vi "PDU Init.vi"(8 "error in (no error)":errorcluster, 10 "Name":string, 11 "Orion PDU in":refnum<class "Orion PDU.lvclass">) -> (0 "error out":errorcluster, 3 "Orion PDU out":refnum<class "Orion PDU.lvclass">)   [LabVIEW 2022 SP3, in "Orion PDU.lvclass"]
uses:
  Orion PDU.lvclass
  C:/Development/rimas/RIMAS/Power Distribution/Power Distribution.lvclass
  Power Distribution.lvclass/Power Distribution.ctl
  Orion PDU.lvclass/Orion PDU.ctl
  Power Distribution.lvclass
  <vilib>/httpClient/LabVIEWHTTPClient.lvlib
panel:
  # "rimas pdu1"
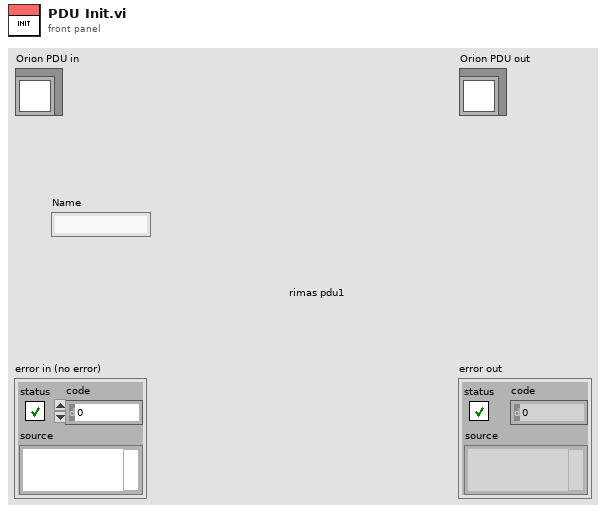
[diagram p1: front panel]
types:
  T1 = typedef "Orion PDU.lvclass/typedef Orion PDU Settings.ctl" = cluster{"URL":string, "Username":string, "Password":string}
  T2 = typedef "LabVIEWHTTPClient.lvlib/ClientHandle.ctl" = refnum<k1>
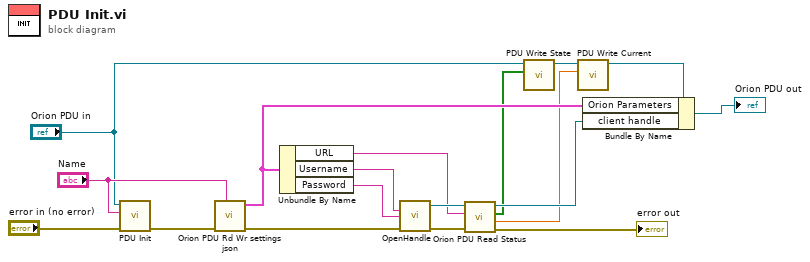
[diagram p0: block diagram]
diagram:
  n1 = call-parent "PDU Init.vi"("error in (no error)"="error in (no error)", "Name"="Name", "Power Distribution in"="Orion PDU in") -> ("error out"=w17:errorcluster)  [unwired: 7 in, 1 out]
  n2 = call "Orion PDU Rd Wr settings json.vi"("Name"="Name", "error in (no error)"=w17) -> ("error out"=w14:errorcluster, "Orion Parameters"=w13:T1)  [unwired: 8 in]
  n3 = Unbundle By Name(w13) -> ("URL"=w8:string, "Username"=w12:string, "Password"=w11:string)
  n4 = call <vilib>:"OpenHandle.vi"("username"=w12, "password"=w11, "error in (no error)"=w14) -> ("client handle out"=w9:T2, "error out"=w10:errorcluster)  [unwired: 11 in]
  n5 = call "Orion PDU Read Status.vi"("error in (no error)"=w10, "Address"=w8, "client handle"=w9) -> ("error out"=→"error out":errorcluster, "current"=w2:dbl, "states"=w6:bool[], "client handle out"=w7:T2)  [unwired: 5 in]
  n6 = call "PDU Write State.vi"("State"=w6, "Power Distribution in"="Orion PDU in") -> ("Power Distribution out"=w4:refnum<class "Orion PDU.lvclass">)  [unwired: 8 in, 1 out]
  n7 = call "PDU Write Current.vi"("Current"=w2, "Power Distribution in"=w4) -> ("Power Distribution out"=w3:refnum<class "Orion PDU.lvclass">)  [unwired: 8 in, 1 out]
  n8 = Bundle By Name(cluster=w3, "Orion Parameters"=w13, "client handle"=w7) -> (→"Orion PDU out":refnum<class "Orion PDU.lvclass">)
